vi "redirect IP addresses.vi"(11 "all":T1[](array[typedef])) -> (1 "valid?":bool, 2 "originals":T1[](array[typedef]), 3 "new":T1[](array[typedef]))   [LabVIEW 2013, in "Scan Engine editor node.lvclass"]
uses:
  Scan Engine editor node.lvclass
  table line.ctl
  <vilib>/NI/Tag Bus Module Framework/channel/TBM channel.lvclass
  <vilib>/NI/Tag Bus/tag/tag descriptor.lvclass/tag descriptor.ctl
  <vilib>/NI/Tag Bus/tag/tag descriptor.lvclass
panel:
  in  "New IP Address":string
  in  "Listbox":i32[](listbox)
  in  "OK Button":bool
  in  "Cancel Button":bool
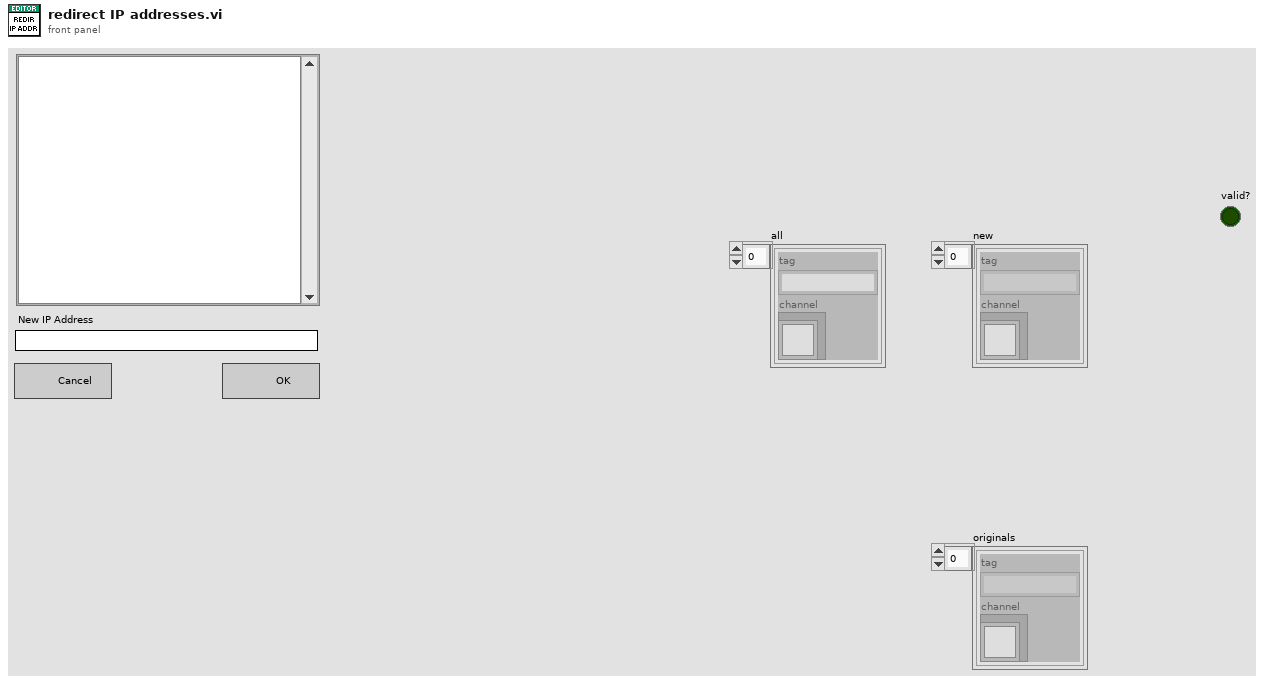
[diagram p1: front panel]
types:
  T1 = typedef "Scan Engine editor node.lvclass/table line.ctl" = cluster{"tag":string, "channel":refnum<class "TBM channel.lvclass">}
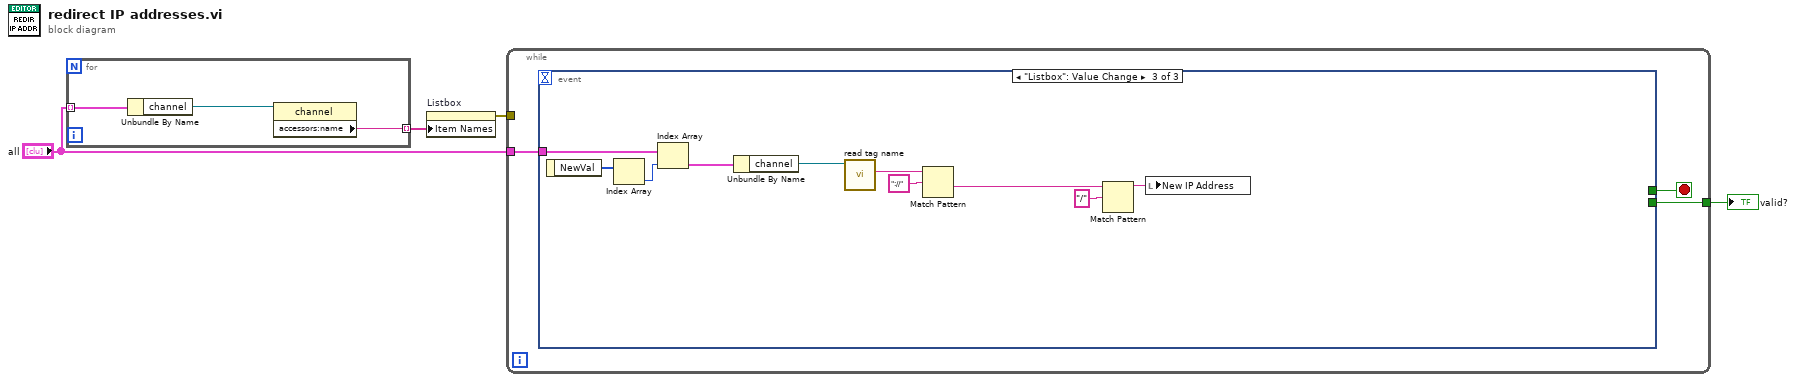
[diagram p0: block diagram]
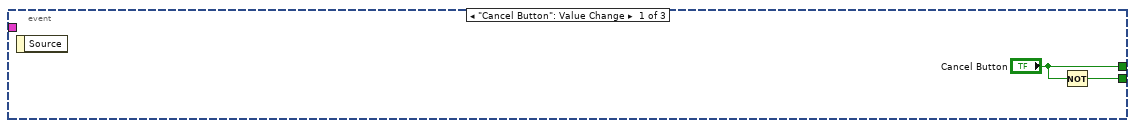
[diagram p2: hidden frame]
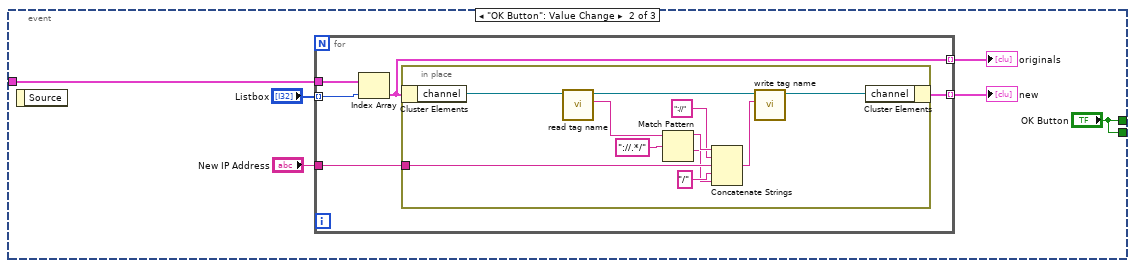
[diagram p3: hidden frame]
diagram:
  n1 = for {
    tunnel: "all" -> [w7] mode=indexing
    tunnel: [w5] -> w4 mode=indexing
    n2 = Unbundle By Name(w7) -> ("channel"=w6:refnum<class "TBM channel.lvclass">)
    n3 = property class="channel"(reference=w6) -> ("accessors:name"=w5:string)  [unwired: 1 in, 2 out]
  }
  n4 = property on="Listbox" class="LstBox (strict)"("Item Names"=w4) -> (error out=w3:errorcluster)  [unwired: 2 in, 1 out]
  n5 = while {
    tunnel: w3 -> [_]
    tunnel: [w9] -> w2
    tunnel: "all" -> [w8]
    stop <- w10 stop-if-true
    n6 = event shown="[2] \"Listbox\": Value Change" {
      selector: _ -> [_ _ _]
      dyn-events: _ -> [_ _ _]
      timeout: _ -> [_ _ _]
      tunnel: ["Cancel Button" "OK Button" _] -> w10
      tunnel: [w12 "OK Button" _] -> w9
      tunnel: w8 -> [_ w16 w43]
      event "Cancel Button": Value Change {
        n7 = event-data() -> ()  [unwired: 1 in, 1 out]
        n8 = Not(x="Cancel Button") -> (.not. x?=w12:bool)
      }
      event "OK Button": Value Change {
        n9 = event-data() -> ()  [unwired: 1 in, 1 out]
        n10 = for {
          tunnel: "Listbox" -> [w23] mode=indexing
          tunnel: w16 -> [w22]
          tunnel: [w21] -> w15 mode=indexing
          tunnel: [w20] -> w14 mode=indexing
          tunnel: "New IP Address" -> [w19]
          n11 = Index Array(array=w22, index=w23) -> (element=w21:T1)
          n12 = in-place {
            in-place-border: w19 -> [w31]
            n13 = in-place-cluster #1(w21) -> ("channel"=w26:refnum<class "TBM channel.lvclass">)
            n14 = call <vilib>:"read tag name.vi"("system tag in"=w26) -> ("name"=w24:string, "system tag out"=w25:refnum<class "TBM channel.lvclass">)  [unwired: 8 in, 1 out]
            n15 = Match Pattern(string=w24, regular expression="://.*/") -> (before substring=w33:string, after substring=w29:string)  [unwired: 1 in, 2 out]
            n16 = Concatenate Strings(w33, "://" ("string"), w31, "/" ("string"), w29) -> (w28:string)
            n17 = call <vilib>:"write tag name.vi"("name"=w28, "system tag in"=w25) -> ("system tag out"=w27:refnum<class "TBM channel.lvclass">)  [unwired: 8 in, 1 out]
            n18 = in-place-cluster #1("channel"=w27) -> (w20:T1)
          }
        }
        "originals" <- w15
        "new" <- w14
      }
      event "Listbox": Value Change {
        n19 = event-data() -> ("NewVal"=w44:i32[])  [unwired: 1 in]
        n20 = Index Array(array=w44) -> (element=w42:i32)  [unwired: 1 in]
        n21 = Index Array(array=w43, index=w42) -> (element=w41:T1)
        n22 = Unbundle By Name(w41) -> ("channel"=w36:refnum<class "TBM channel.lvclass">)
        n23 = call <vilib>:"read tag name.vi"("system tag in"=w36) -> ("name"=w35:string)  [unwired: 8 in, 2 out]
        n24 = Match Pattern(string=w35, regular expression="://") -> (after substring=w39:string)  [unwired: 1 in, 3 out]
        n25 = Match Pattern(string=w39, regular expression="/") -> (before substring=w37:string)  [unwired: 1 in, 3 out]
        n26 = local write "New IP Address"(w37) -> ()
      }
    }
  }
  "valid?" <- w2
